vi "AVG1DScans.vi"() -> ()   [LabVIEW 2022 SP3]
uses:
  <vilib>/Analysis/baseanly.llb/Mean (DBL).vi
  <vilib>/Utility/file.llb/Read From Spreadsheet File (DBL).vi
  <vilib>/Utility/file.llb/Write To Spreadsheet File (DBL).vi
  <vilib>/Analysis/NI_AALBase.lvlib
panel:
  in  "directory path":path
  out "XY Graph":cluster{dbl[], dbl[]}(graph)
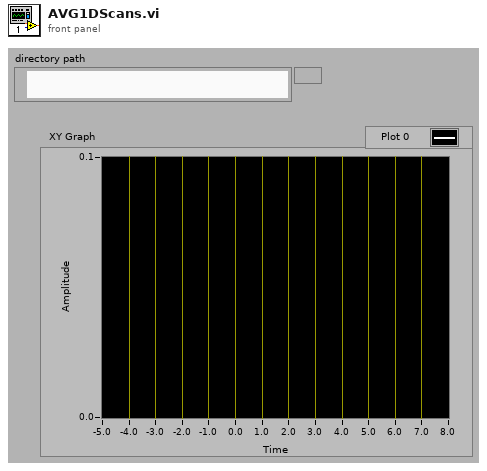
[diagram p1: front panel]
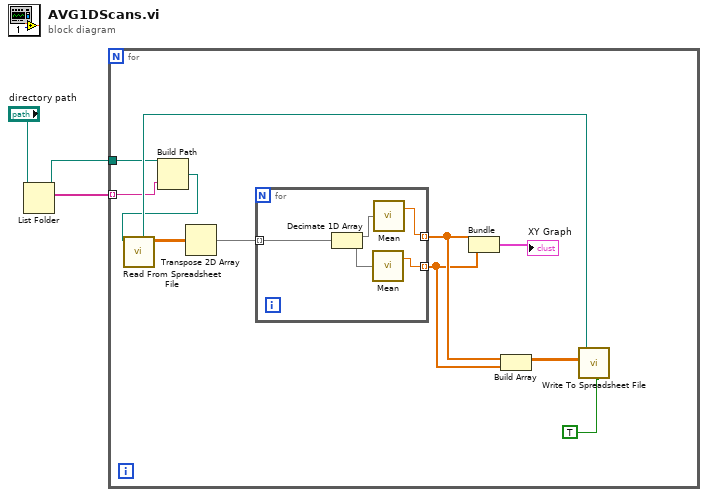
[diagram p0: block diagram]
diagram:
  n1 = List Folder(path="directory path") -> (path out=w2:path, filenames=w3:string[])  [unwired: 1 in, 4 out]
  n2 = for {
    tunnel: w3 -> [w5] mode=indexing
    tunnel: w2 -> [w6]
    n3 = Build Path(base path=w6, name or relative path=w5) -> (appended path=w4:path)
    n4 = call-poly <vilib>:"Read From Spreadsheet File.vi"("file path (dialog if empty)"=w4) -> ("all rows"=w14:dbl[][], "new file path (Not A Path if cancelled)"=w7:path)  [unwired: 3 in, 6 out]
    n5 = Transpose 2D Array(2D array=w14) -> (transposed array=w13:dbl[][])
    n6 = for {
      tunnel: w13 -> [w19] mode=indexing
      tunnel: [w15] -> w11 mode=indexing
      tunnel: [w17] -> w10 mode=indexing
      n7 = Decimate 1D Array(w19) -> (w16:dbl[], w18:dbl[])
      n8 = call-poly <vilib>:"Mean.vi"("X"=w18) -> ("mean"=w17:dbl)  [unwired: 1 out]
      n9 = call-poly <vilib>:"Mean.vi"("X"=w16) -> ("mean"=w15:dbl)  [unwired: 1 out]
    }
    n10 = Bundle(w11, w10) -> (→"XY Graph":cluster{dbl[], dbl[]})  [unwired: 1 out]
    n11 = Build Array(w11, w10) -> (w9:dbl[][])
    n12 = call-poly <vilib>:"Write To Spreadsheet File.vi"("transpose? (no:F)"=TRUE, "2D data"=w9, "file path (dialog if empty)"=w7) -> ()  [unwired: 3 in, 3 out]
  }
